vi "Example.vi"(8 "error in (no error)":errorcluster) -> (0 "error out":errorcluster)   [LabVIEW 2018]
uses:
  <instrlib>/niDMM/nidmm.llb/niDMM Function.ctl
  <instrlib>/niDMM/nidmm.llb/niDMM Resolution in Digits.ctl
  <instrlib>/niDCPower/nidcpower.llb/niDCPower Source Mode.ctl
  <instrlib>/niDCPower/nidcpower.llb/niDCPower Output Function.ctl
  <instrlib>/niDMM/nidmm.llb/niDMM Configure Measurement Digits.vi
  Power_Supply/Power_Supply Virtual/Power_Supply Virtual.lvclass
  DMM/DMM Virtual/DMM Virtual.lvclass
panel:
  out "Meas CH1 (Volts)":dbl format="%_7p"
  out "Meas CH0 (Volts)":dbl format="%_7p"
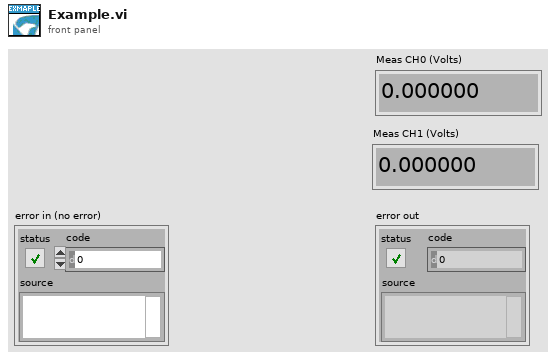
[diagram p1: front panel]
types:
  T1 = typedef "Class Attributes Cluster.ctl" = cluster{"Model Number":string, "Instrument Number":u8, "Rack ID":string, "Inst Mnemonic":string, "Comp Mnemonic":string, "Subsys Mnemonic":string, "IP Address":string, "Sub Address":string, "Firmware Rev":string, "Expected Options":string, "Required Options":string, "Excluded Options":string}
  T2 = typedef "niDMM Function.ctl" = enum16{"DC Volts", "AC Volts", "DC Current", "AC Current", "2-wire Resistance", "4-wire Resistance", "Diode", "Frequency", "Period", "AC Volts DC Coupled", "Capacitance", "Inductance", "Temperature"}
  T3 = typedef "niDCPower Output Function.ctl" = i32
  T4 = typedef "niDCPower Source Mode.ctl" = i32
  T5 = typedef "niDMM Resolution in Digits.ctl" = dbl
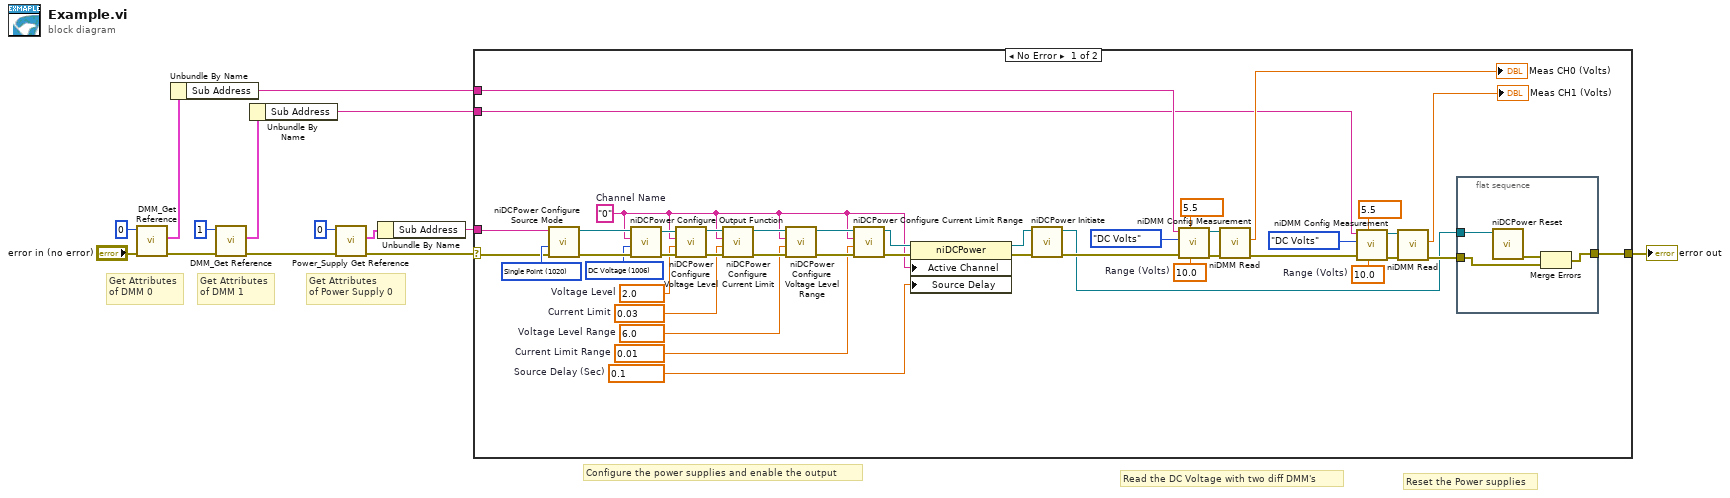
[diagram p0: block diagram]
diagram:
  # "Reset the Power supplies"
  # "Read the DC Voltage with two diff DMM's"
  # "Configure the power supplies and enable the output"
  # "Get Attributes\nof DMM 1"
  # "Get Attributes\nof DMM 0"
  # "Get Attributes\nof Power Supply 0"
  n1 = call "DMM_Get Reference.vi"("error in (no error)"="error in (no error)", "Instrument Reference"=u8 0) -> ("error out"=w2:errorcluster, "Class Attributes"=w1:T1)  [unwired: 7 in, 1 out]
  n2 = Unbundle By Name(w1) -> ("Sub Address"=w9:string)
  n3 = call "DMM_Get Reference.vi"("error in (no error)"=w2, "Instrument Reference"=u8 1) -> ("error out"=w4:errorcluster, "Class Attributes"=w3:T1)  [unwired: 7 in, 1 out]
  n4 = Unbundle By Name(w3) -> ("Sub Address"=w8:string)
  n5 = call "Power_Supply Get Reference.vi"("error in (no error)"=w4, "Instrument Reference"=u8 0) -> ("error out"=w5:errorcluster, "Class Attributes"=w6:T1)  [unwired: 7 in, 1 out]
  n6 = Unbundle By Name(w6) -> ("Sub Address"=w11:string)
  n7 = case shown="No Error" w5 {
    selector: w5 -> [w38 w62]
    tunnel: w11 -> [w37 _]
    tunnel: w9 -> [w51 _]
    tunnel: w8 -> [w43 _]
    tunnel: [w41 w62] -> w7
    frame No Error {
      w16 = "0"  # Channel Name
      w20 = 0.1  # Source Delay (Sec)
      w23 = 0.01  # Current Limit Range
      w24 = 6.0  # Voltage Level Range
      w29 = 0.03  # Current Limit
      w15 = 2.0  # Voltage Level
      w17 = T3 1006 items=["DC Voltage"=1006, "DC Current"=1007, "Pulse Voltage"=1049, "Pulse Current"=1050] ("output function")
      w40 = T4 1020 items=["Single Point"=1020, "Sequence"=1021] ("source mode")
      w50 = T5 5.5 items=["3 1/2"=3.5, "4 1/2"=4.5, "5 1/2"=5.5, "6 1/2"=6.5, "7 1/2"=7.5] ("Resolution in Digits")
      w45 = 10.0  # Range (Volts)
      w52 = T5 5.5 items=["3 1/2"=3.5, "4 1/2"=4.5, "5 1/2"=5.5, "6 1/2"=6.5, "7 1/2"=7.5] ("Resolution in Digits")
      w57 = 10.0  # Range (Volts)
      n8 = call <instrlib>:"niDCPower Configure Source Mode.vi"("error in (no error)"=w38, "source mode"=w40, "instrument handle"=w37) -> ("error out"=w39:errorcluster, "instrument handle out"=w36:refnum<k15>)  [unwired: 7 out]
      n9 = call <instrlib>:"niDCPower Configure Output Function.vi"("error in (no error)"=w39, "output function"=w17, "channel name"=w16, "instrument handle"=w36) -> ("error out"=w18:errorcluster, "instrument handle out"=w19:refnum<k15>)  [unwired: 6 out]
      n10 = call <instrlib>:"niDCPower Configure Voltage Level.vi"("error in (no error)"=w18, "voltage level"=w15, "channel name"=w16, "instrument handle"=w19) -> ("error out"=w30:errorcluster, "instrument handle out"=w31:refnum<k15>)  [unwired: 6 out]
      n11 = call <instrlib>:"niDCPower Configure Current Limit.vi"("error in (no error)"=w30, "current limit"=w29, "channel name"=w16, "instrument handle"=w31) -> ("error out"=w28:errorcluster, "instrument handle out"=w27:refnum<k15>)  [unwired: 1 in, 5 out]
      n12 = call <instrlib>:"niDCPower Configure Voltage Level Range.vi"("error in (no error)"=w28, "voltage level range"=w24, "channel name"=w16, "instrument handle"=w27) -> ("error out"=w26:errorcluster, "instrument handle out"=w25:refnum<k15>)  [unwired: 6 out]
      n13 = call <instrlib>:"niDCPower Configure Current Limit Range.vi"("error in (no error)"=w26, "current limit range"=w23, "channel name"=w16, "instrument handle"=w25) -> ("error out"=w21:errorcluster, "instrument handle out"=w22:refnum<k15>)  [unwired: 6 out]
      n14 = property class="niDCPower"(reference=w22, error in=w21, "Active Channel"=w16, "Source Delay"=w20) -> (reference out=w32:refnum<k15>, error out=w35:errorcluster)
      n15 = call <instrlib>:"niDCPower Initiate.vi"("error in (no error)"=w35, "instrument handle"=w32) -> ("error out"=w34:errorcluster, "instrument handle out"=w33:refnum<k15>)  [unwired: 2 in, 6 out]
      n16 = call-poly <instrlib>:"niDMM Config Measurement.vi"("Range"=w57, "Resolution in Digits"=w52, "error in (no error)"=w34, "Function"=niDMM_Function."DC Volts" ("Measurement Type"), "instrument handle"=w51) -> ("error out"=w54:errorcluster, "instrument handle out"=w53:refnum<k15>)  [unwired: 5 in]
      n17 = call <instrlib>:"niDMM Read.vi"("error in (no error)"=w54, "instrument handle"=w53) -> ("error out"=w44:errorcluster, "Measurement"=→"Meas CH0 (Volts)":dbl)  [unwired: 7 in, 1 out]
      n18 = call-poly <instrlib>:"niDMM Config Measurement.vi"("Range"=w45, "Resolution in Digits"=w50, "error in (no error)"=w44, "Function"=niDMM_Function."DC Volts" ("Measurement Type"), "instrument handle"=w43) -> ("error out"=w48:errorcluster, "instrument handle out"=w49:refnum<k15>)  [unwired: 5 in]
      n19 = call <instrlib>:"niDMM Read.vi"("error in (no error)"=w48, "instrument handle"=w49) -> ("error out"=w42:errorcluster, "Measurement"=→"Meas CH1 (Volts)":dbl)  [unwired: 7 in, 1 out]
      n20 = flat-sequence {
        tunnel: w42 -> [w59]
        tunnel: w33 -> [w61]
        tunnel: [w58] -> w41
        frame #0 {
          n21 = call <instrlib>:"niDCPower Reset.vi"("instrument handle"=w61) -> ("error out"=w60:errorcluster)  [unwired: 3 in, 7 out]
          n22 = Merge Errors(w60, w59) -> (w58:errorcluster)
        }
      }
    }
    frame Error {
    }
  }
  "error out" <- w7
